vi "ep_Compensate Operate Time.vi"(9 "operate time":dbl, 10 "multiples of pickup":dbl, 11 "operate time compensation":cluster{"G/Gs":dbl[], "compensation [s]":dbl[]}) -> (3 "compensated operate time":dbl)   [LabVIEW 2012, in "NI_EP_Protection.lvlib"]
uses:
  <vilib>/addons/Electrical Power/Protection/NI_EP_Protection.lvlib
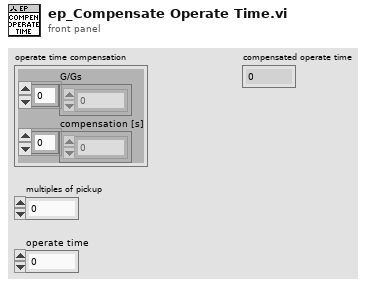
[diagram p1: front panel]
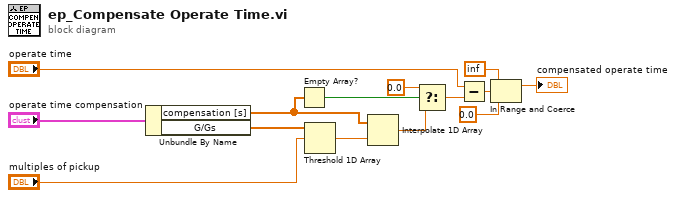
[diagram p0: block diagram]
diagram:
  n1 = Unbundle By Name("operate time compensation") -> ("compensation [s]"=w4:dbl[], "G/Gs"=w3:dbl[])
  n2 = Empty Array?(array=w4) -> (empty?=w6:bool)
  n3 = Threshold 1D Array(2:"multiples of pickup", 3:w3) -> (0:w5:dbl)  [unwired: 1 in]
  n4 = Interpolate 1D Array(1:w5, 2:w4) -> (0:w7:dbl)
  n5 = Select(t=0.0, s=w6, f=w7) -> (s? t:f=w8:dbl)
  n6 = Subtract(x="operate time", y=w8) -> (x-y=w11:dbl)
  n7 = In Range and Coerce(upper limit=inf, x=w11, lower limit=0.0) -> (coerced(x)=→"compensated operate time":dbl)  [unwired: 1 out]
